vi "Stop Core.vi"(6 "final error code":i32, 11 "WS Client in":refnum<class "WS Client.lvclass">) -> (3 "WS Client out":refnum<class "WS Client.lvclass">)   [LabVIEW 2016, in "WebSocket Networking.lvlib" / "WS Client.lvclass"]
doc: "--\nCopyright © 2017 Composed SystemsI All rights reserved.\n\nAuthor: Jon McBee <jon.mcbee@composed.io>\n\nThis library is provided \"AS IS\" ,WITHOUT WARRANTIES OR\nCONDITIONS OF ANY KIND, either express or implied.\n\nComposed Systems -- composed.io\n\nStream 0.0.1.1\nJon McBee - Composed Systems\nCopyright (c) 2017, Composed Systems"
uses:
  <userlib>/Common Components/WebSocket Networking/WS Client/WS Client.lvclass
  C:/Program Files (x86)/National Instruments/LabVIEW 2016/user.lib/Composed Systems/Stream/Mediator/Classes/Mediated Asynchronous Actor/Mediated Asynchronous Actor.lvclass
  <userlib>/Common Components/WebSocket Networking/WS Client/WS Client.lvclass/WS Client.ctl
  <userlib>/Composed Systems/Stream/Mediator/Classes/Websocket Client Handler Actor/Websocket Client Handler/Websocket Client Handler.lvclass
  <userlib>/Composed Systems/Stream/Mediator/Classes/Mediated Asynchronous Actor/Mediated Asynchronous Actor.lvclass
  <userlib>/Common Components/WebSocket Networking/WS Server Msgs/Remove Connected Client from WSserver Msg/Remove Connected Client from WSserver Msg.lvclass
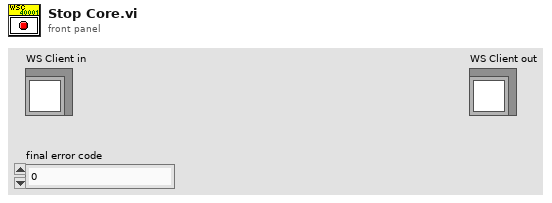
[diagram p1: front panel]
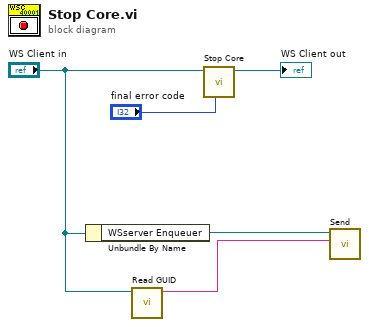
[diagram p0: block diagram]
diagram:
  n1 = Unbundle By Name("WS Client in") -> ("WSserver Enqueuer"=w3:refnum<class "Message Transport Queue.lvclass">)
  n2 = call <userlib>:"Read GUID.vi"("Mediated Asynchronous Actor in"="WS Client in") -> ("GUID"=w2:string)  [unwired: 10 in]
  n3 = call-parent "Stop Core.vi"("final error code"="final error code", "Websocket Client Handler in"="WS Client in") -> ("Websocket Client Handler out"=→"WS Client out":refnum<class "WS Client.lvclass">)  [unwired: 9 in]
  n4 = call <userlib>:"Send.vi"("GUID"=w2, "Message Transport Queue"=w3) -> ()  [unwired: 9 in, 1 out]
